vi "PromptForInputTemplate.vi"() -> ()   [LabVIEW 2018]
uses:
  <vilib>/event_ctls.llb/eventvkey.ctl
panel:
  in  "Cancel":bool
  in  "OK":bool
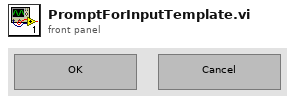
[diagram p1: front panel]
types:
  T1 = typedef "eventvkey.ctl" = enum16{"ASCII", "Enter", "Return", "Shift", "Ctrl", "Alt", "Cmd", "Opt", "Caps", "NumLock", "Clear", "Break", "Up", "Down", "Left", "Right", "Insert", "Delete", "Home", "End", "PageUp", "PageDown", "Escape", "Help", "Pause", "ScrollLock", "F1", "F2", "F3", "F4", "F5", "F6", "F7", "F8", "F9", "F10", "F11", "F12", "F13", "F14", "F15", "F16", "F17", "F18", "F19", "F20", "F21", "F22", "F23", "F24", "Play", "VolumeUp", "VolumeDown", "Mute", "Two Byte Char"}
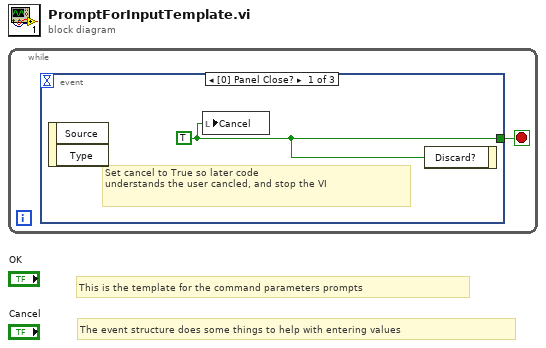
[diagram p0: block diagram]
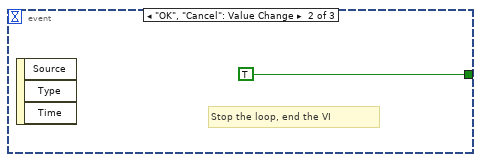
[diagram p2: hidden frame]
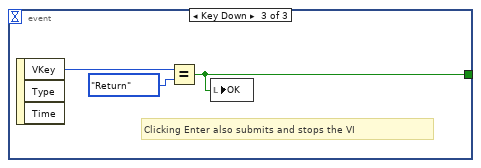
[diagram p3: hidden frame]
diagram:
  # "The event structure does some things to help with entering values"
  # "This is the template for the command parameters prompts"
  n1 = while {
    stop <- w1 stop-if-true
    n2 = event shown="[0] Panel Close?" {
      selector: _ -> [_ _ _]
      dyn-events: _ -> [_ _ _]
      timeout: _ -> [_ _ _]
      tunnel: [w2 TRUE ("Discard?") w4] -> w1
      event Panel Close? {
        w2 = TRUE ("Discard?")
        # "Set cancel to True so later code\nunderstands the user cancled, and stop the VI"
        n3 = event-data() -> ()  [unwired: 1 in, 2 out]
        n4 = local write "Cancel"(w2) -> ()
        n5 = event-data("Discard?"=w2) -> ()  [unwired: 1 in, 1 out]
      }
      event "OK", "Cancel": Value Change {
        # "Stop the loop, end the VI"
        n6 = event-data() -> ()  [unwired: 1 in, 3 out]
      }
      event Key Down {
        # "Clicking Enter also submits and stops the VI"
        n7 = event-data() -> ("VKey"=w6:T1)  [unwired: 1 in, 2 out]
        n8 = Equal?(x=w6, y=eventvkey."Return") -> (x = y?=w4:bool)
        n9 = local write "OK"(w4) -> ()
      }
    }
  }
